vi "Edge Detection Hatch V2.vi"(7 "error in":errorcluster) -> (27 "error out":errorcluster)   [LabVIEW 2018]
uses:
  <vilib>/vision/driver/IMAQdx.llb/IMAQdx Camera Control Mode.ctl
  <vilib>/userdefined/High Color/IMAQdx.ctl
  <vilib>/vision/Measure.llb/Edge Options.ctl
  <vilib>/vision/Measure.llb/Edge Polarity.ctl
  <vilib>/vision/Measure.llb/Straight Edge Options.ctl
  <vilib>/vision/Measure.llb/Straight Edge Process.ctl
  <vilib>/Analysis/baseanly.llb/Mean (DBL).vi
  <vilib>/Analysis/1siggen.llb/Ramp Pattern by Delta.vi
  <vilib>/vision/NI_Vision_Development_Module.lvlib
  <vilib>/vision/driver/NI_Vision_Acquisition_Software.lvlib
  <resource>/objmgr/imaqdx.rc
  <vilib>/Analysis/NI_AALBase.lvlib
  <vilib>/ptbypt/NI_PtbyPt.lvlib
panel:
  out "Image Out 3":T1(plugin-control)
  out "element 2":T2
  out "mean":dbl format="%0.2f"
  in  "stop":bool
  out "XY Graph":cluster{"Ramp Pattern":dbl[], u32[]}(graph)
  out "Centerpoint 4":cluster{dbl, dbl}
  out "Particle Reports (Pixels)":T3(array[cluster]) {"Orientation" format="%.2f"; "Dimensions"."Height" format="%.2f"; "Dimensions"."Width" format="%.2f"; "Center of Mass"."Y" format="%.2f"; "Center of Mass"."X" format="%.2f"; "Bounding Rect"."Bottom" format="%.2f"; "Bounding Rect"."Right" format="%.2f"; "Bounding Rect"."Top" format="%.2f"; "Bounding Rect"."Left" format="%.2f"; "Number of Holes" format="%.2f"; "Area" format="%.2f"}
  out "Centerpoint 3":cluster{dbl, dbl}
  out "Merged Centerpoint":cluster{dbl, dbl}
  out "Image Out 2":T1(plugin-control)
  in  "error in 3":errorcluster
  in  "error in 2":errorcluster
  out "Run time":u32
  out "Image Out":T1(plugin-control)
types:
  T1 = typedef "IMAQ Image.ctl" = refnum<image>
  T2 = cluster{"Area":dbl, "Number of Holes":dbl, "Bounding Rect":cluster{"Left":dbl, "Top":dbl, "Right":dbl, "Bottom":dbl}, "Center of Mass":cluster{"X":dbl, "Y":dbl}, "Orientation":dbl, "Dimensions":cluster{"Width":dbl, "Height":dbl}}
  T3 = cluster{"Area":dbl, "Number of Holes":dbl, "Bounding Rect":cluster{"Left":dbl, "Top":dbl, "Right":dbl, "Bottom":dbl}, "Center of Mass":cluster{"X":dbl, "Y":dbl}, "Orientation":dbl, "Dimensions":cluster{"Width":dbl, "Height":dbl}}[]
  T4 = typedef "IMAQdx.ctl" = refnum<k21>
  T5 = typedef "NI_Vision_Acquisition_Software.lvlib/IMAQdx Camera Control Mode.ctl" = enum32{"Controller", "Listener"}
  T6 = typedef "Image Type" = u32
  T7 = cluster{"Measurement Parameter":i32, "Range Lower Value":dbl, "Range Upper Value":dbl, "Range":bool, "Measurement Type":bool}[]
  T8 = enum32{"AutoM", "Close", "Dilate", "Erode", "Gradient", "Gradient out", "Gradient in", "Hit miss", "Open", "PClose", "POpen", "Thick", "Thin"}
  T9 = typedef "Particle Parameters" = i32
  T10 = cluster{"Measurement Parameter":T9, "Range Lower Value":dbl, "Range Upper Value":dbl, "Range":bool, "Measurement Type":bool}[]
  T11 = cluster{"Brightness":sgl, "Contrast":sgl, "Gamma":sgl}
  T12 = typedef "ROI Descriptor" = cluster{"Global Rectangle":i32[], "Contours":cluster{"ID":enum32{"External", "Internal"}, "Type":u32, "Coordinates":i32[]}[]}
  T13 = cluster{"histogram":u32[], "Minimal Value":sgl, "Maximal Value":sgl, "Starting Value":sgl, "Interval Width":sgl, "Mean Value":sgl, "Standard  Variation":sgl, "Area (pixels)":i32}
  T14 = typedef "Straight Edge Options.ctl" = cluster{"Number of Lines":i32, "Type":T15, "Min. Score":dbl, "Max. Score":dbl, "Orientation":dbl, "Angle Range":dbl, "Angle Tolerance":dbl, "Step Size":u32, "Min. SNR (db)":dbl, "Min. Points (%)":dbl, "Hough Iterations":i32}
  T15 = typedef "Straight Edge Process.ctl" = enum32{"First Edge Rake", "Best Edge Rake", "Hough Edge Rake", "First Edge Projection", "Best Edge Projection"}
  T16 = typedef "Edge Options.ctl" = cluster{"Edge Polarity":T17, "Kernel Size":u32, "Width":u32, "Minimum Edge Strength":sgl, "Interpolation Type":enum32{"Zero Order", "Bilinear", "Quadratic", "Cubic", "Bilinear Fixed"}, "Data Processing Method":enum32{"Average", "Median"}}
  T17 = typedef "Edge Polarity.ctl" = u32
  T18 = typedef "Search Line.ctl" = cluster{"Start Point":cluster{"X":sgl, "Y":sgl}, "End Point":cluster{"X":sgl, "Y":sgl}, "Edge Info":T19[], "Edge Map":dbl[], "Calibration Valid":bool}
  T19 = typedef "Edge New.ctl" = cluster{"Location (Pixel)":cluster{"X":sgl, "Y":sgl}, "Location (Real-World)":cluster{"X":sgl, "Y":sgl}, "Distance (Pixel)":dbl, "Distance (Real-World)":dbl, "Strength":dbl, "Noise":dbl, "Rising?":bool}
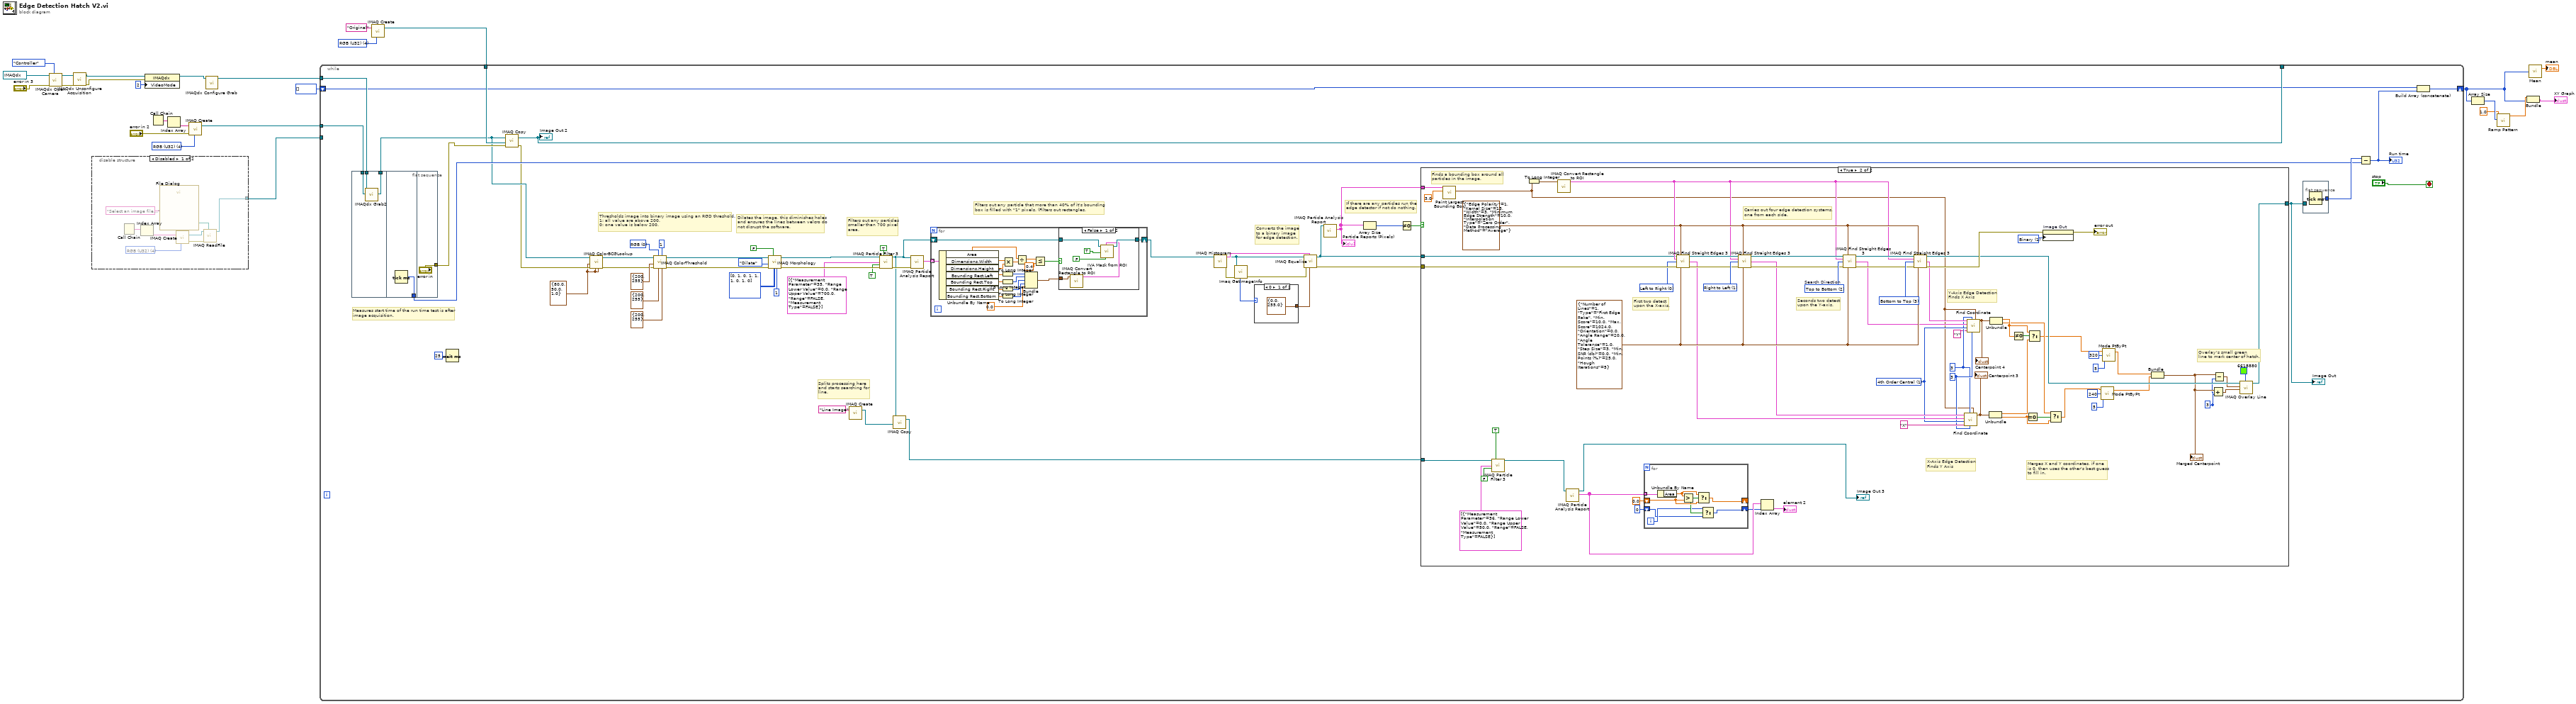
[diagram p0: block diagram]
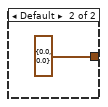
[diagram p5: hidden frame]
diagram:
  w11 = T6 4 items=["Grayscale (U8)", "Grayscale (I16)", "Grayscale (SGL)", "Complex (CSG)", "RGB (U32)", "HSL (U32)", "RGB (U64)", "Grayscale (U16)"] ("Image Type")
  w26 = T6 4 items=["Grayscale (U8)", "Grayscale (I16)", "Grayscale (SGL)", "Complex (CSG)", "RGB (U32)", "HSL (U32)", "RGB (U64)", "Grayscale (U16)"] ("Image Type")
  n1 = call <vilib>:"IMAQdx Open Camera.vi"("Camera Control Mode"=IMAQdx_Camera_Control_Mode."Controller", "error in"="error in 3", "Session In"=T4 "cam1") -> ("error out"=w17:errorcluster, "Session Out"=w18:T4)  [unwired: 7 in]
  n2 = call <vilib>:"IMAQdx Unconfigure Acquisition.vi"("error in"=w17, "Session In"=w18) -> ("error out"=w20:errorcluster, "Session Out"=w19:T4)  [unwired: 8 in]
  n3 = disable-structure shown="Disabled" {
    disable-tunnel: [w27 _] -> w21
    frame Disabled {
      w28 = T6 4 items=["Grayscale (U8)", "Grayscale (I16)", "Grayscale (SGL)", "Complex (CSG)", "RGB (U32)", "HSL (U32)", "RGB (U64)", "Grayscale (U16)"] ("Image Type")
      n4 = Call Chain() -> (call chain=w31:string[])
      n5 = Index Array(array=w31) -> (element=w32:string)  [unwired: 1 in]
      n6 = call "File Dialog"("prompt"="Select an image file...") -> ("selected path"=w33:path)  [unwired: 6 in, 8 out]
      n7 = call "IMAQ Create"("Image Name"=w32, "Image Type"=w28) -> ("New Image"=w29:T1, "error out"=w30:errorcluster)  [unwired: 2 in, 1 out]
      n8 = call "IMAQ ReadFile"("File Path"=w33, "error in (no error)"=w30, "Image"=w29) -> ("Image Out"=w27:T1)  [unwired: 2 in, 6 out]
    }
    frame Enabled {
    }
  }
  n9 = property class="IMAQdx"(reference=w19, error in=w20, "VideoMode"=u32 2) -> (reference out=w16:T4)  [unwired: 1 out]
  n10 = Call Chain() -> (call chain=w13:string[])
  n11 = Index Array(array=w13) -> (element=w12:string)  [unwired: 1 in]
  n12 = call "IMAQ Create"("Image Name"=w12, "Image Type"=w11, "error in (no error)"="error in 2") -> ("New Image"=w23:T1)  [unwired: 1 in, 2 out]
  n13 = call <vilib>:"IMAQdx Configure Grab.vi"("Session In"=w16) -> ("Session Out"=w22:T4)  [unwired: 9 in, 1 out]
  n14 = call "IMAQ Create"("Image Name"="Original", "Image Type"=w26) -> ("New Image"=w24:T1)  [unwired: 2 in, 2 out]
  n15 = while {
    tunnel: w24 -> [w61]
    tunnel: [w56] -> _
    tunnel: w23 -> [w55]
    tunnel: w22 -> [w54]
    tunnel: w21 -> [_]
    shift-right: [w47] -> w2
    shift-left: u32[] [] -> [w46]
    stop <- "stop" stop-if-true
    w40 = T11 {"Brightness"=80.0, "Contrast"=50.0, "Gamma"=1.0} ("Green BCG Values")
    w84 = u16 0 items=["RGB", "HSL", "HSV", "HSI"] ("Color Mode")
    # "Splits processing here\nand starts searching for\nline."
    # "If there are any particles run the \nedge detector if not do nothing."
    # "Converts the image\nto a binary image\nfor edge detection."
    # "Filters out any particle that more than 40% of it's bounding \nbox is filled with \"1\" pixels. (Filters out rectangles."
    # "Filters out any particles\nsmaller than 700 pixel\narea."
    # "Dilates the image, this diminishes holes \nand ensures the lines between velcro do\nnot disrupt the software."
    # "Thresholds image into binary image using an RGD threshold.\n1: all value are above 200.\n0: one value is below 200."
    # "Measures start time of the run time test is after\nimage acquisition."
    n16 = flat-sequence {
      tunnel: w55 -> [w89]
      tunnel: w54 -> [w88]
      tunnel: [w87] -> w44
      tunnel: [w90] -> w63
      tunnel: ["error in"] -> w59
      frame #0 {
        n17 = call <vilib>:"IMAQdx Grab2.vi"("Image In"=w89, "Session In"=w88) -> ("Image Out"=w87:T1)  [unwired: 6 in, 3 out]
      }
      frame #1 {
        n18 = Tick Count (ms)() -> (millisecond timer value=w90:u32)
      }
      frame #2 {
      }
    }
    n19 = Wait (ms)(milliseconds to wait=u32 25) -> ()  [unwired: 1 out]
    n20 = call "IMAQ Copy"("error in (no error)"=w59, "Image Dst"=w61, "Image Src"=w44) -> ("error out"=w42:errorcluster, "Image Dst Out"=w56:T1)  [unwired: 3 in]
    "Image Out 2" <- w56
    n21 = call "IMAQ ColorBCGLookup"("Blue BCG Values"=w40, "Green BCG Values"=w40, "error in (no error)"=w42, "Red BCG Values"=w40, "Image Src"=w44) -> ("error out"=w41:errorcluster, "Image Dst Out"=w43:T1)  [unwired: 2 in, 3 out]
    n22 = call "IMAQ ColorThreshold"("Blue or Luma or Val or Inten Range"=cluster{"Lower value":i32, "Upper value":i32} {"Lower value"=200, "Upper value"=255}, "Replace Value"=1, "Green or Sat Range"=cluster{"Lower value":i32, "Upper value":i32} {"Lower value"=200, "Upper value"=255}, "Color Mode"=w84, "error in (no error)"=w41, "Red or Hue Range"=cluster{"Lower value":i32, "Upper value":i32} {"Lower value"=200, "Upper value"=255}, "Image Src"=w43) -> ("error out"=w80:errorcluster, "Image Dst Out"=w75:T1)  [unwired: 1 in, 2 out]
    n23 = call "IMAQ Morphology"("Number of iterations (1)"=1, "Structuring Element"=i32[][] [[0, 1, 0], [1, 1, 1], [0, 1, 0]], "Square/Hexa (Square)"=FALSE, "error in (no error)"=w80, "Operation"=T8."Dilate", "Image Src"=w75) -> ("error out"=w74:errorcluster, "Image Dst Out"=w71:T1)  [unwired: 1 in, 3 out]
    n24 = call "IMAQ Create"("Image Name"="Line Image") -> ("New Image"=w36:T1)  [unwired: 4 in, 1 out]
    n25 = call "IMAQ Particle Filter 3"("Image Src"=w71, "Connectivity 4/8 (8)"=TRUE, "Selection Values"=T7 [{"Measurement Parameter"=35, "Range Lower Value"=0.0, "Range Upper Value"=700.0, "Range"=FALSE, "Measurement Type"=FALSE}], "Keep/Remove Particles (F)"=TRUE ("Keep/Remove Particles"), "error in (no error)"=w74) -> ("Image Dst Out"=w37:T1, "error out"=w60:errorcluster)  [unwired: 4 in, 5 out]
    n26 = call "IMAQ Copy"("Image Dst"=w36, "Image Src"=w37) -> ("Image Dst Out"=w35:T1)  [unwired: 4 in, 1 out]
    n27 = call "IMAQ Particle Analysis Report"("error in (no error)"=w60, "Image"=w37) -> ("Particle Reports (Pixels)"=w57:T3)  [unwired: 4 in, 5 out]
    n28 = for {
      tunnel: w57 -> [w185] mode=indexing
      shift-right: [w177] -> w58
      shift-left: w37 -> [w178]
      n29 = Unbundle By Name(w185) -> ("Area"=w182:dbl, "Dimensions.Width"=w184:dbl, "Dimensions.Height"=w183:dbl, "Bounding Rect.Left"=w175:dbl, "Bounding Rect.Top"=w174:dbl, "Bounding Rect.Right"=w173:dbl, "Bounding Rect.Bottom"=w172:dbl)
      n30 = To Long Integer(number=w175) -> (32bit integer=w171:i32)
      n31 = To Long Integer(number=w174) -> (32bit integer=w170:i32)
      n32 = To Long Integer(number=w173) -> (32bit integer=w169:i32)
      n33 = To Long Integer(number=w172) -> (32bit integer=w168:i32)
      n34 = Multiply(x=w184, y=w183) -> (x*y=w181:dbl)
      n35 = Divide(x=w182, y=w181) -> (x/y=w180:dbl)
      n36 = Bundle(w171, w170, w169, w168, 0.0) -> (w167:cluster{i32, i32, i32, i32, dbl})  [unwired: 1 in]
      n37 = Less Or Equal?(x=w180, y=0.4) -> (x <= y?=w176:bool)
      n38 = case shown="False" w176 {
        tunnel: w178 -> [w188 w192]
        tunnel: [w187 w192] -> w177
        tunnel: w167 -> [w191 _]
        frame False {
          n39 = call "IMAQ Convert Rectangle to ROI"("Rectangle"=w191) -> ("ROI Descriptor"=w186:T12)  [unwired: 8 in, 1 out]
          n40 = call <vilib>:"IVA Mask from ROI.vi"("Shrink"=FALSE, "ROI Descriptor"=w186, "Out / In"=TRUE, "Image Src"=w188) -> ("Image Out"=w187:T1)  [unwired: 1 in, 6 out]
        }
        frame True {
        }
      }
    }
    n41 = call "IMAQ Histogram"("Image"=w58) -> ("error out"=w67:errorcluster, "Histogram Report"=w69:T13)  [unwired: 4 in, 5 out]
    n42 = call "Imaq GetImageInfo"("error in (no error)"=w67, "Image"=w58) -> ("error out"=w66:errorcluster, "Image Type"=w68:T6)  [unwired: 8 out]
    n43 = case shown="0" w68 {
      tunnel: [cluster{"Minimum":sgl, "Maximum":sgl} {"Minimum"=0.0, "Maximum"=255.0} ("Range") cluster{"Minimum":sgl, "Maximum":sgl} {"Minimum"=0.0, "Maximum"=0.0} ("Range")] -> w65
      frame 0 {
      }
      frame Default {
      }
    }
    n44 = call "IMAQ Equalize"("Range"=w65, "Histogram Report"=w69, "error in (no error)"=w66, "Image Src"=w58) -> ("error out"=w52:errorcluster, "Image Dst Out"=w53:T1)  [unwired: 2 in, 4 out]
    n45 = call "IMAQ Particle Analysis Report"("Image"=w53) -> ("Particle Reports (Pixels)"=w51:T3)  [unwired: 5 in, 5 out]
    "Particle Reports (Pixels)" <- w51
    n46 = Array Size(array=w51) -> (size(s)=w50:i32)
    n47 = Not Equal To 0?(x=w50) -> (x != 0?=w49:bool)
    n48 = case shown="True" w49 {
      tunnel: w51 -> [_ w150]
      tunnel: [w92 w145] -> w48
      tunnel: w53 -> [w92 w101]
      tunnel: w52 -> [_ w140]
      tunnel: w35 -> [_ w93]
      frame False {
      }
      frame True {
        w115 = 3
        w125 = 3 ("Subset Length")
        w126 = 3 ("Detector Interval")
        w135 = u32 0 items=["Left to Right", "Right to Left", "Top to Bottom", "Bottom to Top"] ("Search Direction")
        w142 = u32 1 items=["Left to Right", "Right to Left", "Top to Bottom", "Bottom to Top"] ("Search Direction")
        w137 = T14 {"Number of Lines"=1, "Type"=enum."First Edge Rake", "Min. Score"=10.0, "Max. Score"=1024.0, "Orientation"=0.0, "Angle Range"=20.0, "Angle Tolerance"=1.0, "Step Size"=3, "Min. SNR (db)"=0.0, "Min. Points (%)"=25.0, "Hough Iterations"=5} ("Line Options")
        w138 = T16 {"Edge Polarity"=1, "Kernel Size"=13, "Width"=3, "Minimum Edge Strength"=10.0, "Interpolation Type"=enum."Zero Order", "Data Processing Method"=enum."Average"} ("Edge Options")
        w128 = u16 1 items=["2nd Order Central", "4th Order Central", "Forward", "Backward"] ("method")
        w152 = u32 3 items=["Left to Right", "Right to Left", "Top to Bottom", "Bottom to Top"] ("Search Direction")
        w155 = u32 1 items=["Grayscale", "Binary", "Gradient", "Rainbow", "Temperature", "User Defined", "Binary 16 Bit", "Gradient 16 Bit", "Rainbow 16 Bit", "Temperature 16 Bit", "User Defined 16 Bit"] ("Palette Type")
        w157 = u32 2 items=["Left to Right", "Right to Left", "Top to Bottom", "Bottom to Top"]  # Search Direction
        # "Merges X and Y coordinates, if one\nis 0, then uses the other's best guess \nto fill in."
        # "Overlay's small green\nline to mark center of hatch."
        # "Seconds two detect\nupon the Y-axis."
        # "First two detect\nupon the X-axis."
        # "Carries out four edge detection systems,\none from each side."
        # "Finds a bounding box around all\nparticles in the image."
        # "Y-Axis Edge Detection\nFinds X Axis"
        # "X-Axis Edge Detection\nFinds Y Axis"
        n49 = call "Paint Largest Bounding Box.vi"("Border Width"=3.0, "Particle Reports (Pixels)"=w150) -> ("Bounding Box"=w124:cluster{dbl, dbl, dbl, dbl, dbl})  [unwired: 8 in, 1 out]
        n50 = call "IMAQ Particle Filter 3"("Image Src"=w93, "Connectivity 4/8 (8)"=TRUE, "Selection Values"=T10 [{"Measurement Parameter"=36, "Range Lower Value"=0.0, "Range Upper Value"=50.0, "Range"=FALSE, "Measurement Type"=FALSE}], "Keep/Remove Particles (F)"=FALSE ("Keep/Remove Particles")) -> ("Image Dst Out"=w95:T1)  [unwired: 5 in, 6 out]
        n51 = To Long Integer(number=w124) -> (32bit integer=w154:cluster{i32, i32, i32, i32, i32})
        n52 = call "IMAQ Convert Rectangle to ROI"("Rectangle"=w154) -> ("ROI Descriptor"=w136:T12)  [unwired: 8 in, 1 out]
        n53 = call "IMAQ Particle Analysis Report"("Image"=w95) -> ("Particle Reports (Pixels)"=w98:T3, "Image Out (duplicate)"=→"Image Out 3":T1)  [unwired: 5 in, 4 out]
        n54 = for {
          tunnel: w98 -> [w165] mode=indexing
          shift-right: [w162] -> _
          shift-left: 0.0 ("Area") -> [w163]
          shift-right: [w159] -> w97
          shift-left: 0 -> [w158]
          i -> [w160]
          n55 = Unbundle By Name(w165) -> ("Area"=w164:dbl)
          n56 = Greater?(x=w164, y=w163) -> (0:w161:bool)
          n57 = Select(t=w164, s=w161, f=w163) -> (s? t:f=w162:dbl)
          n58 = Select(t=w160, s=w161, f=w158) -> (s? t:f=w159:i32)
        }
        n59 = call "IMAQ Find Straight Edges 3"("Image"=w101, "Edge Options"=w138, "ROI Descriptor"=w136, "Search Direction"=w135, "error in (no error)"=w140, "Line Options"=w137) -> ("Image (duplicate)"=w141:T1, "Search Lines Information"=w133:T18[], "error out"=w139:errorcluster)  [unwired: 1 in, 6 out]
        n60 = call "IMAQ Find Straight Edges 3"("Image"=w141, "Edge Options"=w138, "ROI Descriptor"=w136, "Search Direction"=w142, "error in (no error)"=w139, "Line Options"=w137) -> ("Image (duplicate)"=w144:T1, "Search Lines Information"=w134:T18[], "error out"=w143:errorcluster)  [unwired: 1 in, 6 out]
        n61 = Index Array(array=w98, index=w97) -> (element=→"element 2":T2)
        n62 = call "IMAQ Find Straight Edges 3"("Image"=w144, "Edge Options"=w138, "ROI Descriptor"=w136, "Search Direction"=w157, "error in (no error)"=w143, "Line Options"=w137) -> ("Image (duplicate)"=w151:T1, "Search Lines Information"=w129:T18[], "error out"=w148:errorcluster)  [unwired: 1 in, 6 out]
        n63 = call "IMAQ Find Straight Edges 3"("Image"=w151, "Edge Options"=w138, "ROI Descriptor"=w136, "Search Direction"=w152, "error in (no error)"=w148, "Line Options"=w137) -> ("Image (duplicate)"=w146:T1, "Search Lines Information"=w130:T18[], "error out"=w153:errorcluster)  [unwired: 1 in, 6 out]
        n64 = call "Find Coordinate.vi"("Bounding Box"=w124, "Detector Interval"=w126, "Subset Length"=w125, "String"="X", "method"=w128, "Search Lines Information 2"=w133, "Search Lines Information"=w134) -> ("Centerpoint 3"=w131:cluster{dbl, dbl})  [unwired: 4 in]
        "Centerpoint 3" <- w131
        n65 = call "Find Coordinate.vi"("Bounding Box"=w124, "Detector Interval"=w126, "Subset Length"=w125, "String"="Y", "method"=w128, "Search Lines Information 2"=w129, "Search Lines Information"=w130) -> ("Centerpoint 3"=w127:cluster{dbl, dbl})  [unwired: 4 in]
        "Centerpoint 4" <- w127
        n66 = Unbundle(w131) -> (w121:dbl, w118:dbl)
        n67 = Unbundle(w127) -> (w122:dbl, w119:dbl)
        n68 = Not Equal To 0?(x=w122) -> (x != 0?=w123:bool)
        n69 = Equal To 0?(x=w118) -> (x = 0?=w120:bool)
        n70 = Select(t=w122, s=w123, f=w121) -> (s? t:f=w112:dbl)
        n71 = property on="Image Out" class="ImageControl"(error in=w153, "Palette:Palette Type"=w155) -> (error out=→"error out":errorcluster)  [unwired: 1 in, 1 out]
        n72 = Select(t=w119, s=w120, f=w118) -> (s? t:f=w106:dbl)
        n73 = call <vilib>:"Mode PtByPt.vi"("sample length"=5, "intervals"=240, "x"=w106) -> ("mode"=w105:dbl)  [unwired: 1 in, 1 out]
        n74 = call <vilib>:"Mode PtByPt.vi"("sample length"=5, "intervals"=320, "x"=w112) -> ("mode"=w109:dbl)  [unwired: 1 in, 1 out]
        n75 = Bundle("mode"=w109, "mode"=w105) -> (w116:cluster{"mode":dbl, "mode":dbl})  [unwired: 1 in]
        "Merged Centerpoint" <- w116
        n76 = Add(x=w116, y=w115) -> (x+y=w117:cluster{"mode":dbl, "mode":dbl})
        n77 = Subtract(x=w116, y=w115) -> (x-y=w114:cluster{"mode":dbl, "mode":dbl})
        n78 = call "IMAQ Overlay Line"("Color"=u32 6618880, "End Point"=w117, "Start Point"=w114, "Image"=w146) -> ("Image Out"=w145:T1)  [unwired: 6 in, 1 out]
      }
    }
    "Image Out" <- w48
    n79 = flat-sequence {
      tunnel: [w86] -> w64
      tunnel: w48 -> [_]
      frame #0 {
        n80 = Tick Count (ms)() -> (millisecond timer value=w86:u32)
      }
    }
    n81 = Subtract(x=w64, y=w63) -> (x-y=w45:u32)
    "Run time" <- w45
    n82 = Build Array (concatenate)(w46, w45) -> (w47:u32[])
  }
  n83 = Array Size(array=w2) -> (size(s)=w6:i32)
  n84 = call-poly <vilib>:"Ramp Pattern.vi"("end"=w6, "delta"=1.0) -> ("Ramp Pattern"=w4:dbl[])  [unwired: 7 in, 2 out]
  n85 = Bundle("Ramp Pattern"=w4, w2) -> (→"XY Graph":cluster{"Ramp Pattern":dbl[], u32[]})  [unwired: 1 in]
  n86 = call-poly <vilib>:"Mean.vi"("X"=w2) -> ("mean"=→"mean":dbl)  [unwired: 1 out]
